vi "ReadImageSize.vi"(8 "error in":errorcluster, 11 "Image Reference In":T1) -> (0 "error out":errorcluster, 1 "Height":i32, 2 "Width":i32, 3 "Image Reference Out":T1)   [LabVIEW 2024, in "OpenLvVision_Image.lvlib" / "Management.lvlib"]
doc: "Returns the image dimensions in pixel."
uses:
  TypeDef/Image.ctl
  Management.lvlib
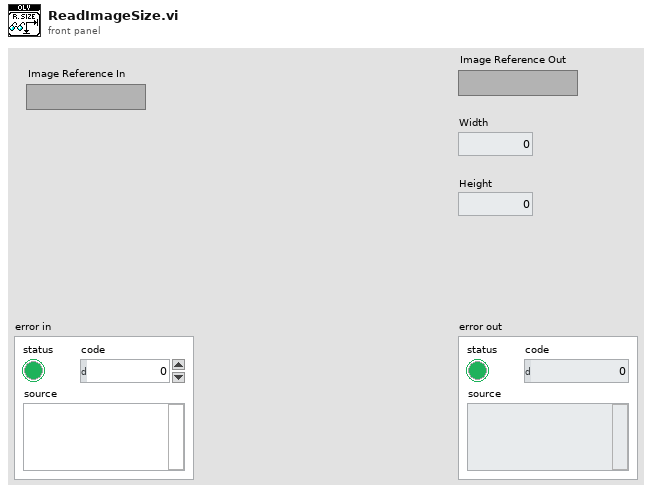
[diagram p1: front panel]
types:
  T1 = typedef "OpenLvVision_Image.lvlib/Management.lvlib/Image.ctl" = refnum<image>
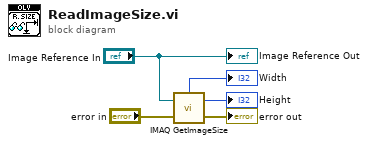
[diagram p0: block diagram]
diagram:
  n1 = call "IMAQ GetImageSize"("Image"="Image Reference In", "error in (no error)"="error in") -> ("Y Resolution"=→"Height":i32, "X Resolution"=→"Width":i32, "error out"=→"error out":errorcluster)  [unwired: 2 in]
  "Image Reference Out" <- "Image Reference In"
